vi "Disabled - Split Array (SubVI).vi"(6 "Force Reload":bool, 9 "all rows":dbl[][](array[numeric]), 11 "File Name":string="test.pi") -> (3 "Auto Array":dbl[][](array[numeric]))   [LabVIEW 2017]
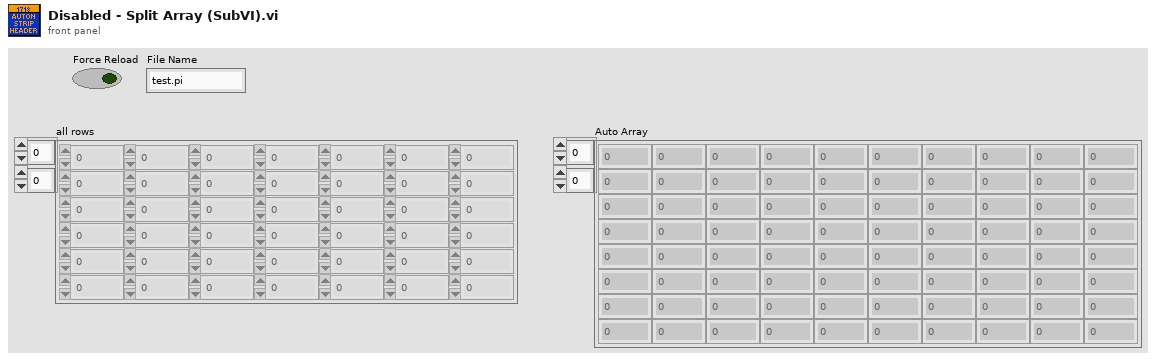
[diagram p1: front panel]
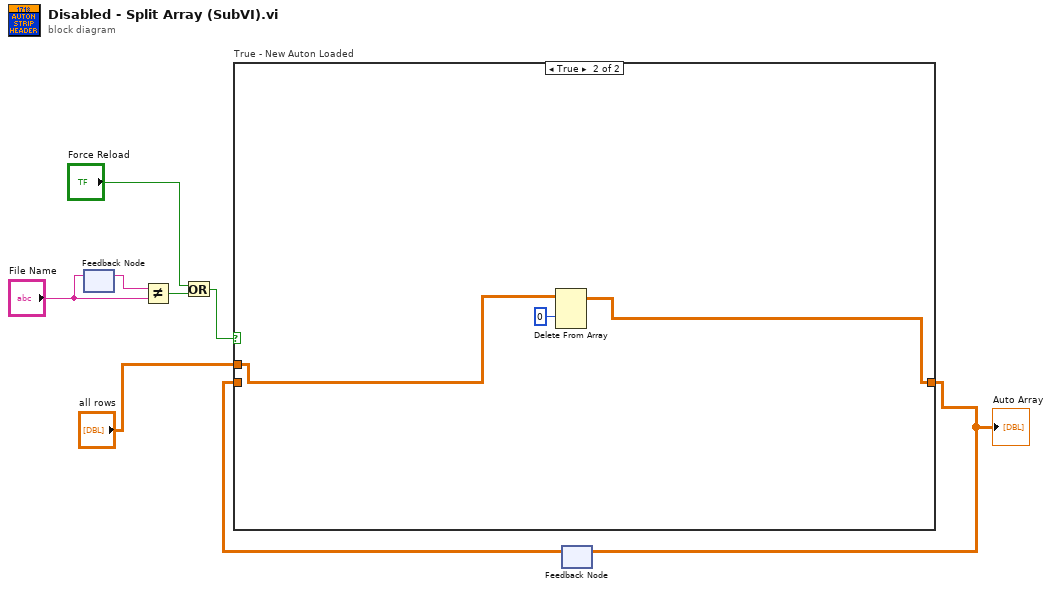
[diagram p0: block diagram]
diagram:
  n1 = feedback-in #1("File Name") -> ()
  n2 = feedback #1() -> (w6:string)  [unwired: 1 in]
  n3 = Not Equal?(x=w6, y="File Name") -> (x != y?=w5:bool)
  n4 = Or(x="Force Reload", y=w5) -> (x .or. y?=w3:bool)
  n5 = feedback #2() -> (w8:dbl[][])  [unwired: 1 in]
  n6 = case "True - New Auton Loaded" shown="True" w3 {
    tunnel: [w9 w10] -> w1
    tunnel: w8 -> [w9 _]
    tunnel: "all rows" -> [_ w12]
    frame False {
    }
    frame True {
      n7 = Delete From Array(array=w12, index (row)=0) -> (array with subset deleted=w10:dbl[][])  [unwired: 2 in, 1 out]
    }
  }
  "Auto Array" <- w1
  n8 = feedback-in #2(w1) -> ()
